vi "Get Measurement Details.vi"(8 "error in":errorcluster) -> (0 "error out":errorcluster, 1 "measurement annotations":T1[](array[typedef]), 2 "service class":string, 3 "measurement details":T2)   [LabVIEW 2021, in "Scalar Efficiency And Load Regulation_PMIC.lvlib"]
uses:
  Scalar Efficiency And Load Regulation_PMIC.lvlib
  <vilib>/Plug-In SDKs/Measurements/Helpers/TypeDefs/Measurement Details.ctl
  <vilib>/Plug-In SDKs/Measurements/Helpers/TypeDefs/Measurement Annotation.ctl
  <vilib>/Plug-In SDKs/Measurements/NI Measurement Plug-In SDK.lvlib
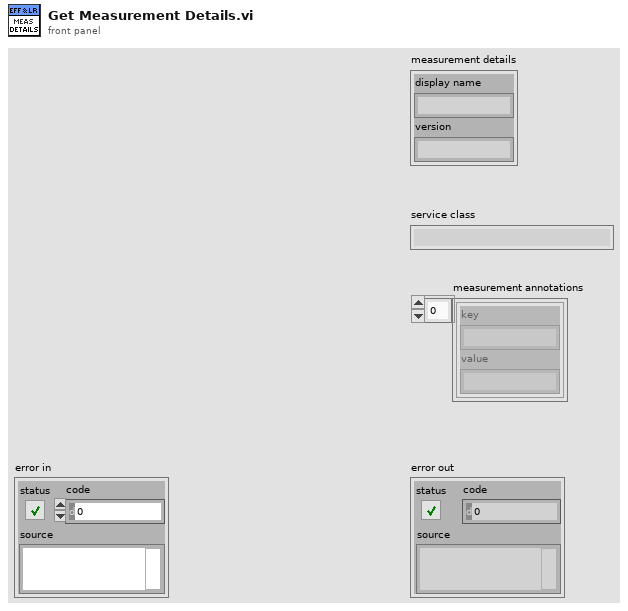
[diagram p1: front panel]
types:
  T1 = typedef "NI Measurement Plug-In SDK.lvlib/Measurement Annotation.ctl" = cluster{"key":string, "value":string}
  T2 = typedef "NI Measurement Plug-In SDK.lvlib/Measurement Details.ctl" = cluster{"display name":string, "version":string}
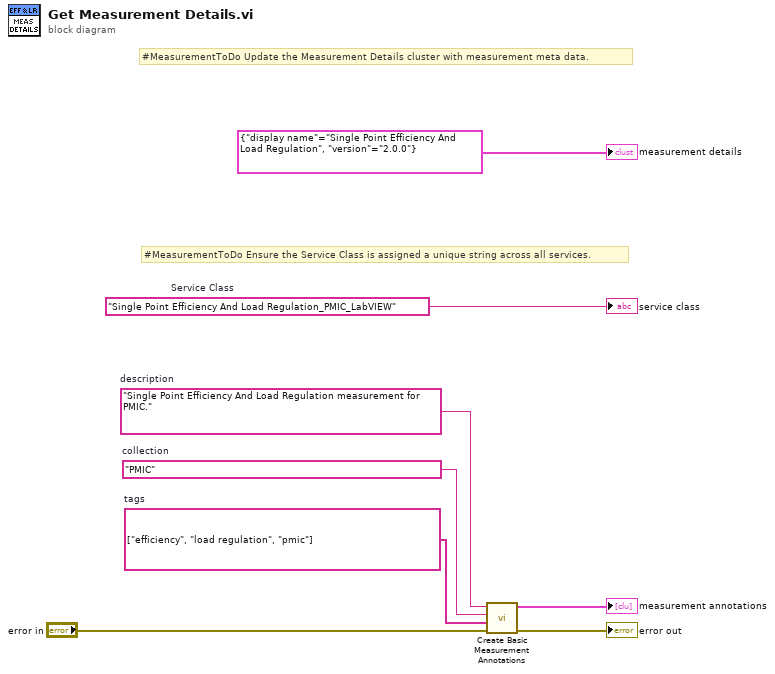
[diagram p0: block diagram]
diagram:
  w1 = "Single Point Efficiency And Load Regulation measurement for PMIC."  # description
  w2 = string[] ["efficiency", "load regulation", "pmic"]  # tags
  w3 = "PMIC"  # collection
  w8 = "Single Point Efficiency And Load Regulation_PMIC_LabVIEW"  # Service Class
  # "#MeasurementToDo Ensure the Service Class is assigned a unique string across all services."
  # "#MeasurementToDo Update the Measurement Details cluster with measurement meta data."
  n1 = call <vilib>:"Create Basic Measurement Annotations.vi"("error in"="error in", "tags"=w2, "collection"=w3, "description"=w1) -> ("error out"=→"error out":errorcluster, "measurement annotations"=→"measurement annotations":T1[])  [unwired: 6 in]
  "measurement details" <- T2 {"display name"="Single Point Efficiency And Load Regulation", "version"="2.0.0"} ("Measurement Details")
  "service class" <- w8
